vi "Overlay LineOut.vi"(6 "Font, Size & Style":T1={"Desired Font (Application)"=enum."Application Font", "[User-specified Font]"={"Font Name"="", "Size"=12, "Strikeout?"=FALSE, "Italic?"=FALSE, "Underline?"=FALSE, "Outline?"=FALSE, "Shadow?"=FALSE, "Bold?"=FALSE, "Rotation Angle"=0.0}, "Horizontal Alignment"=0, "Vertical Alignment"=0} {"Vertical Alignment" items=["Bottom", "Top", "Baseline"]; "Horizontal Alignment" items=["Left", "Center", "Right"]; "[User-specified Font]"."Rotation Angle" format="%.2f"}, 7 "Group":string, 8 "error in":errorcluster, 9 "LineCoord":i32[](array[numeric]), 10 "Calibration":dbl[unit]=1e-06, 11 "Image In":T2) -> (0 "error out":errorcluster, 1 "Image Out":T2, 2 "FWHM":dbl, 3 "Line Graph":cluster{"x0":sgl, "dx":sgl, "Pixels Line":sgl[]})   [LabVIEW 2014, in "POLARIS Vision utility.lvlib"]
doc: "creates overlay poligon line for a trend. If slope of the line is les 45° trend appears at bottom border otherwise at the left border. \n\nthanks for idee and first implementation to Sebastian Keppler, FSU-IOQ\n\nauthor: Alexander Kessler, Helmholtz-Institut-Jena \nmaintainer: Alexander Kessler: alexander.kessler@uni-jena.de\n\n\n\nLicense Agreement for this software:\n\nCopyright (C)\nHelmholtz-Institut-Jena\nFröbelstieg 3\n07743 Jena\nGermany\n\nThis program is free software; you can redistribute it and/or modify it under the terms of the GNU General Public License as published by the Free Software Foundation; either version 2 of the license, or (at your option) any later version.\n\nThis program is distributed in the hope that it will be useful, but WITHOUT ANY WARRANTY; without even the implied warranty of MERCHANTABILITY or FITNESS FOR A PARTICULAR PURPOSE. See the GNU General License for more details (http://www.gnu.org)."
uses:
  POLARIS Vision utility.lvlib
  <vilib>/vision/Image Controls.llb/IMAQ Image.ctl
  <vilib>/Analysis/1siggen.llb/Ramp Pattern by Samples.vi
  <vilib>/vision/NI_Vision_Development_Module.lvlib
  <vilib>/Analysis/NI_AALBase.lvlib
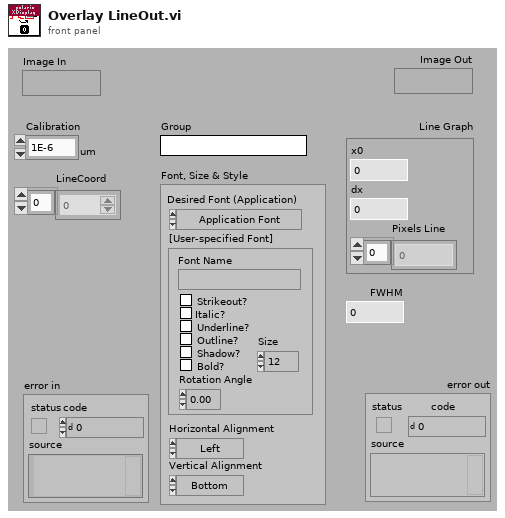
[diagram p1: front panel]
types:
  T1 = cluster{"Desired Font (Application)":enum16{"User-specified Font", "Application Font", "System Font", "Dialog Font"}, "[User-specified Font]":cluster{"Font Name":string, "Size":i16, "Strikeout?":bool, "Italic?":bool, "Underline?":bool, "Outline?":bool, "Shadow?":bool, "Bold?":bool, "Rotation Angle":dbl}, "Horizontal Alignment":i16, "Vertical Alignment":i16}
  T2 = typedef "IMAQ Image.ctl" = refnum<image>
  T3 = cluster{"Min":sgl, "Max":sgl, "Mean":sgl, "Std Dev":sgl, "Count":i32}
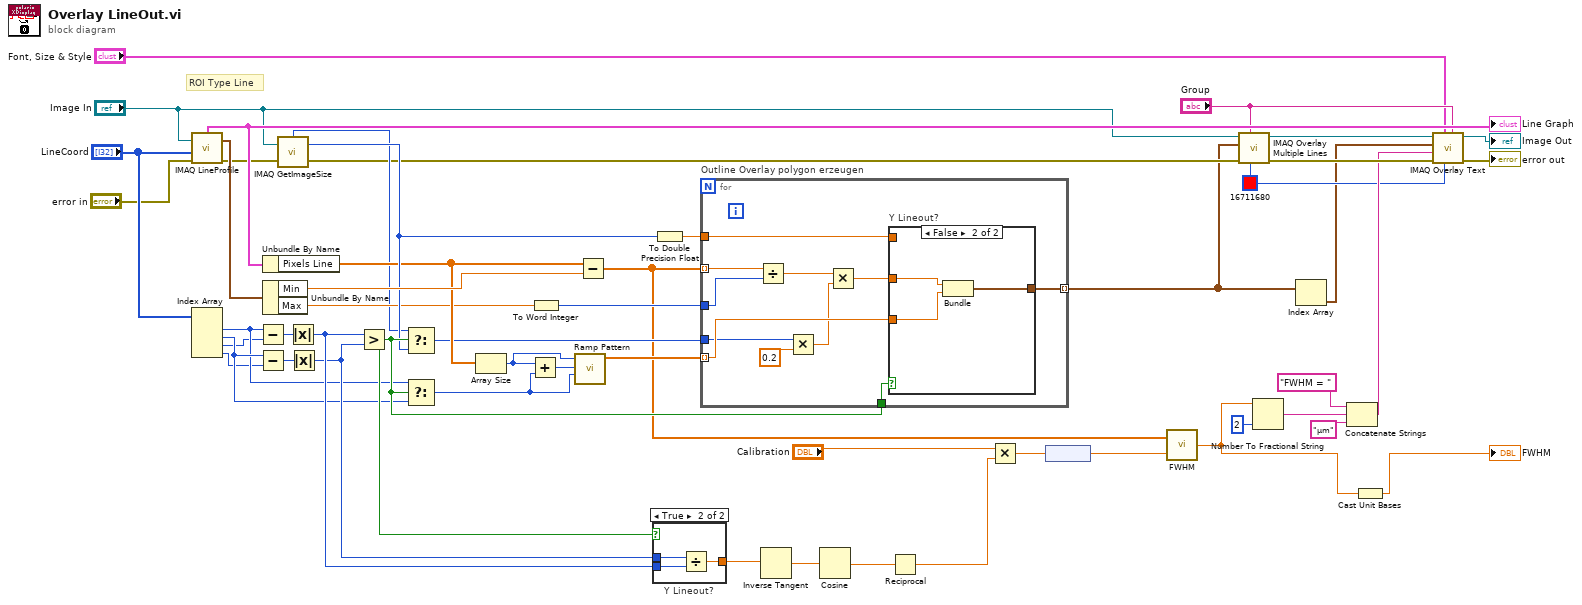
[diagram p0: block diagram]
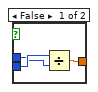
[diagram p2: hidden frame]
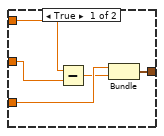
[diagram p3: hidden frame]
diagram:
  w11 = u32 16711680 ("Color")
  # "ROI Type Line"
  n1 = call "IMAQ LineProfile"("error in (no error)"="error in", "Line Coordinates"="LineCoord", "Image"="Image In") -> ("error out"=w26:errorcluster, "Line Graph"=w39:cluster{"x0":sgl, "dx":sgl, "Pixels Line":sgl[]}, "Line Information"=w36:T3)  [unwired: 2 in, 1 out]
  "Line Graph" <- w39
  n2 = Index Array(array="LineCoord") -> (element #1=w44:i32, element #2=w45:i32, element #3=w35:i32, element #4=w30:i32)  [unwired: 4 in]
  n3 = Subtract(x=w44, y=w35) -> (x-y=w31:i32)
  n4 = Subtract(x=w45, y=w30) -> (x-y=w32:i32)
  n5 = Unbundle By Name(w39) -> ("Pixels Line"=w40:sgl[])
  n6 = Unbundle By Name(w36) -> ("Min"=w48:sgl, "Max"=w37:sgl)
  n7 = call "IMAQ GetImageSize"("Image"="Image In", "error in (no error)"=w26) -> ("Y Resolution"=w46:i32, "X Resolution"=w33:i32, "error out"=w27:errorcluster)  [unwired: 2 in]
  n8 = Absolute Value(x=w31) -> (abs(x)=w51:i32)
  n9 = Absolute Value(x=w32) -> (abs(x)=w50:i32)
  n10 = Greater?(x=w51, y=w50) -> (0:w49:bool)
  n11 = Select(t=w33, s=w49, f=w46) -> (s? t:f=w34:i32)
  n12 = Select(t=w44, s=w49, f=w45) -> (s? t:f=w42:i32)
  n13 = Array Size(array=w40) -> (size(s)=w41:i32)
  n14 = Add(x=w41, y=w42) -> (x+y=w43:i32)
  n15 = To Word Integer(number=w37) -> (16bit integer=w38:i16)
  n16 = call-poly <vilib>:"Ramp Pattern.vi"("start"=w42, "end"=w43, "samples"=w41) -> ("Ramp Pattern"=w23:dbl[])  [unwired: 7 in, 1 out]
  n17 = Subtract(x=w40, y=w48) -> (x-y=w10:sgl[])
  n18 = case "Y Lineout?" shown="True" w49 {
    tunnel: w50 -> [w54 w58]
    tunnel: w51 -> [w55 w57]
    tunnel: [w53 w56] -> w14
    frame False {
      n19 = Divide(x=w55, y=w54) -> (x/y=w53:dbl)
    }
    frame True {
      n20 = Divide(x=w58, y=w57) -> (x/y=w56:dbl)
    }
  }
  n21 = To Double Precision Float(number=w46) -> (double precision float=w47:dbl)
  n22 = for "Outline Overlay polygon erzeugen" {
    tunnel: w23 -> [w67] mode=indexing
    tunnel: w10 -> [w66] mode=indexing
    tunnel: [w69] -> w8 mode=indexing
    tunnel: w38 -> [w64]
    tunnel: w34 -> [w62]
    tunnel: w49 -> [w60]
    tunnel: w47 -> [w59]
    n23 = Divide(x=w66, y=w64) -> (x/y=w65:sgl)
    n24 = Multiply(x=w62, y=0.2) -> (x*y=w61:dbl)
    n25 = Multiply(x=w65, y=w61) -> (x*y=w68:dbl)
    n26 = case "Y Lineout?" shown="False" w60 {
      tunnel: [w74 w77] -> w69
      tunnel: w68 -> [w72 w76]
      tunnel: w67 -> [w73 w75]
      tunnel: w59 -> [w70 _]
      frame True {
        n27 = Subtract(x=w70, y=w72) -> (x-y=w71:dbl)
        n28 = Bundle(w73, w71) -> (w74:cluster{dbl, dbl})  [unwired: 1 in]
      }
      frame False {
        n29 = Bundle(w76, w75) -> (w77:cluster{dbl, dbl})  [unwired: 1 in]
      }
    }
  }
  n30 = Inverse Tangent(1:w14) -> (0:w15:dbl)
  n31 = Cosine(x=w15) -> (cos(x)=w13:dbl)
  n32 = Reciprocal(x=w13) -> (1/x=w12:dbl)
  n33 = Multiply(x="Calibration", y=w12) -> (x*y=w3:dbl[unit])
  n34 = node(w3) -> (w2:dbl)
  n35 = call "FWHM.vi"("calibration"=w2, "array"=w10) -> ("FHWM"=w5:dbl)
  n36 = call "IMAQ Overlay Multiple Lines"("Color"=w11, "Group"="Group", "error in (no error)"=w27, "Line End Points"=w8, "Image"="Image In") -> ("error out"=w28:errorcluster, "Image Out"=w24:T2)  [unwired: 5 in]
  n37 = Number To Fractional String(number=w5, precision (6)=i16 2) -> (F-format string=w20:string)  [unwired: 2 in]
  n38 = Index Array(array=w8) -> (element=w7:cluster{dbl, dbl})  [unwired: 1 in]
  n39 = Concatenate Strings("FWHM = " ("string"), w20, "µm" ("string")) -> (w17:string)
  n40 = Cast Unit Bases(0:w5) -> (2:→"FWHM":dbl)  [unwired: 1 in]
  n41 = call "IMAQ Overlay Text"("Group"="Group", "Text Color (black)"=w11, "Font, Size & Style"="Font, Size & Style", "error in (no error)"=w28, "String"=w17, "Origin"=w7, "Image"=w24) -> ("error out"=→"error out":errorcluster, "Image Out"=→"Image Out":T2)  [unwired: 3 in]
